vi "PS35_GoRef.vi"(4 "error in (no error)":errorcluster, 5 "Mode":i32=1 min=0 max=7, 6 "Axis number":i32=1 min=1 max=3, 7 "Control unit ID":i32=1 min=1 max=10) -> (0 "error out":errorcluster)   [LabVIEW 2020]
doc: "PS35_GoRef.vi, created: 04.03.2009 alex; last change: 22.10.2019 alex;\n\n<B>FUNCTION:</B> \n\nDrive an axis to reference.\nReference run is carried out with information of the reference mode. \nThis is valid only for released axes. The suitable reference switch \nshould be configured before. The direction of the reference run is \ndetermined with the speed values (sign).\n----------------------------------------------------------------------------------------\n<B>INPUT:</B>\n[I32] <B>Control unit ID:</B> control unit index. (Default=1, Range=1...10) \n[I32] <B>Axis number:</B> axis number. (Default=1, Range=1...3) \n[I32] <B>Mode:</B> reference mode. (Default=1, Range=0...7) \n0 - search for next index impulse in positive direction and stop\n1 - search for reference switch and release switch\n2 - search for reference switch and next index impulse, then stop\n3 - search for next index impulse (as mode 0) and set counter to zero\n4 - search for reference switch (as mode 1) and set counter to zero\n5 - search for reference switch and next index impulse (as mode 2), \nthen set counter to zero\n6 - search for max. reference switch, search for min. reference switch, \nthen set counter to zero\n7 - search for min. reference switch, search for max. reference switch, \nthen set counter to zero\n[CLU] <B>error in</B>\n----------------------------------------------------------------------------------------\n<B>OUTPUT:</B>\n[CLU] <B>error out</B>\n----------------------------------------------------------------------------------------\n<B>SUB-VIs:</B>\n----------------------------------------------------------------------------------------\n<B>EXT-Calls:</B>\nps35.dll (V2.01)\n----------------------------------------------------------------------------------------"
uses:
  ps35.dll
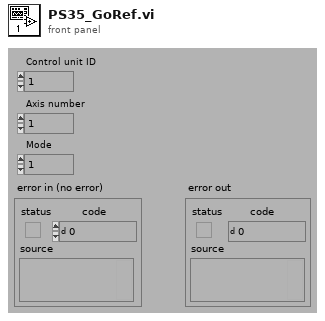
[diagram p1: front panel]
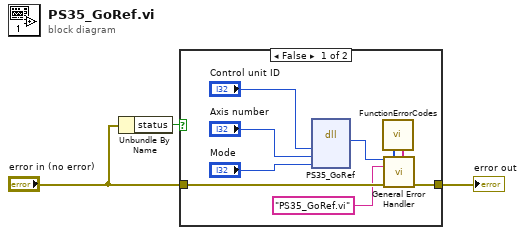
[diagram p0: block diagram]
diagram:
  n1 = Unbundle By Name("error in (no error)") -> ("status"=w1:bool)
  n2 = case shown="False" w1 {
    tunnel: "error in (no error)" -> [w11 w13]
    tunnel: [w10 w13] -> w3
    frame False {
      n3 = dll-call lib="C:/GEECS/Developers Version/source/Device Drivers/OwiSoft/OWISoftOEM/ps35/labview/lv82/ps35.dll" fn="PS35_GoRef"("Index"="Control unit ID", "AxisNr"="Axis number", "Mode"="Mode") -> ("Rückgabetyp"=w9:i32)  [unwired: 6 in, 2 out]
      n4 = call "FunctionErrorCodes.vi"() -> ("[user-defined codes]"=w4:i32[], "[user-defined descriptions]"=w5:string[])  [unwired: 8 in]
      n5 = call <vilib>:"General Error Handler.vi"("[error code] (0)"=w9, "[user-defined codes]"=w4, "[user-defined descriptions]"=w5, "[error source] (\" \")"="PS35_GoRef.vi" ("[error source] (\" \")"), "error in (no error)"=w11) -> ("error out"=w10:errorcluster)  [unwired: 6 in, 4 out]
    }
    frame True {
    }
  }
  "error out" <- w3
